vi "Plug-in test Glimpse version.vi"(7 "Minimum version required":i32) -> (1 "OK?":bool, 3 "Version number":i32)   [LabVIEW 2016]
doc: "Checks whether an appropriate version of Glimpse is loaded.\n\nIntended for non-interactive use only."
uses:
  GLIMPSE Globals.vi
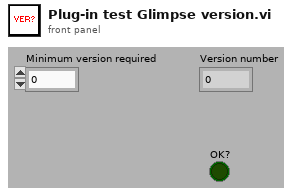
[diagram p1: front panel]
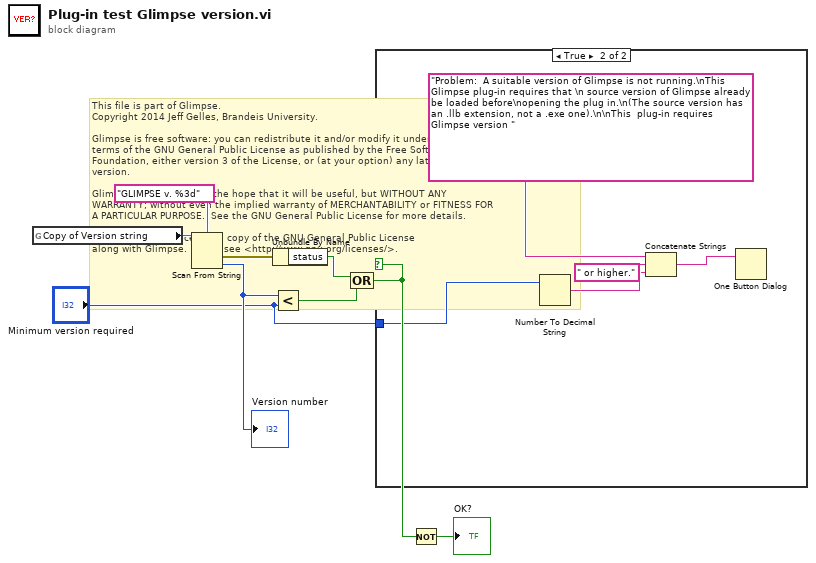
[diagram p0: block diagram]
diagram:
  # "This file is part of Glimpse. \nCopyright 2014 Jeff Gelles, Brandeis University.    \n\nGlimpse is free software: you can redistribute it and/or modify it under the \nterms of the GNU General Public License as published by the Free Software \nFoundation, either version 3 of the License, or (at your option) any later \nversion.\n\nGlimpse is distributed in the hope that it will be useful, but WITHOUT ANY \nWARRANTY; without even the implied warranty of MERCHANTABILITY or FITNESS FOR \nA PARTICULAR PURPOSE.  See the GNU General Public License for more details.\n\nYou should have received a copy of the GNU General Public License\nalong with Glimpse.  If not, see <http://www.gnu.org/licenses/>."
  n1 = global read "GLIMPSE Globals.vi" "Copy of Version string"() -> (w9:string)
  n2 = Scan From String(format string="GLIMPSE v. %3d", input string=w9) -> (error out=w7:errorcluster, output 1=w6:i32)  [unwired: 2 in, 3 out]
  "Version number" <- w6
  n3 = Unbundle By Name(w7) -> ("status"=w5:bool)
  n4 = Less?(x=w6, y="Minimum version required") -> (x < y?=w4:bool)
  n5 = Compound Arithmetic op=OR(w5, w4) -> (w3:bool)
  n6 = case shown="True" w3 {
    tunnel: "Minimum version required" -> [_ w11]
    frame False {
    }
    frame True {
      n7 = Number To Decimal String(number=w11) -> (decimal integer string=w12:string)  [unwired: 1 out]
      n8 = Concatenate Strings("Problem:  A suitable version of Glimpse is not running.\nThis Glimpse plug-in requires that \n source version of Glimpse already be loaded before\nopening the plug in.\n(The source version has an .llb extension, not a .exe one).\n\nThis  plug-in requires Glimpse version " ("message"), w12, " or higher." ("string")) -> (w13:string)
      n9 = One Button Dialog(message=w13) -> ()  [unwired: 2 out]
    }
  }
  n10 = Not(x=w3) -> (.not. x?=→"OK?":bool)
